vi "Add vi to LV Class.vi"(2 "scope":T1(ring)=enum."public", 3 "Error In":errorcluster, 4 "Vi to add to class":string, 5 "Open Library":refnum<vi>) -> (0 "error out":errorcluster, 1 "Open Library":refnum<vi>)   [LabVIEW 2012, in "Scripting Tools.lvlib"]
uses:
  Scripting Tools.lvlib
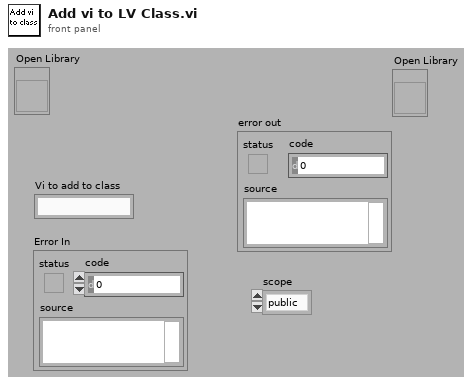
[diagram p1: front panel]
types:
  T1 = enum32{"invalid scope", "public", "private", "protected"}
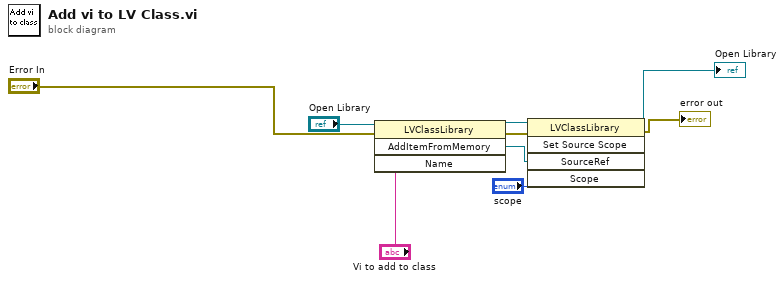
[diagram p0: block diagram]
diagram:
  n1 = invoke class="LVClassLibrary" method="AddItemFromMemory"(reference="Open Library", error in="Error In", "Name"="Vi to add to class") -> (reference out=w6:refnum<vi>, error out=w5:errorcluster, "AddItemFromMemory"=w4:refnum<vi>)  [unwired: 1 in, 1 out]
  n2 = invoke class="LVClassLibrary" method="Set Source Scope"(reference=w6, error in=w5, "SourceRef"=w4, "Scope"="scope") -> (reference out=→"Open Library":refnum<vi>, error out=→"error out":errorcluster)  [unwired: 1 in, 3 out]
